vi "GET.vi"(6 "timeout (10000)":i32=10000, 7 "output file":path=path "", 8 "error in (no error)":errorcluster, 10 "url":string, 11 "HTTP Client Base in":refnum<class "HTTP Client Base.lvclass">) -> (0 "error out":errorcluster, 1 "body":string, 2 "headers":string, 3 "HTTP Client Base out":refnum<class "HTTP Client Base.lvclass">)   [LabVIEW 2021, in "HTTP Client Base.lvclass"]
uses:
  HTTP Client Base.lvclass
  HTTP Client Base.lvclass/HTTP Client Base.ctl
  <vilib>/httpClient/LabVIEWHTTPClient.lvlib
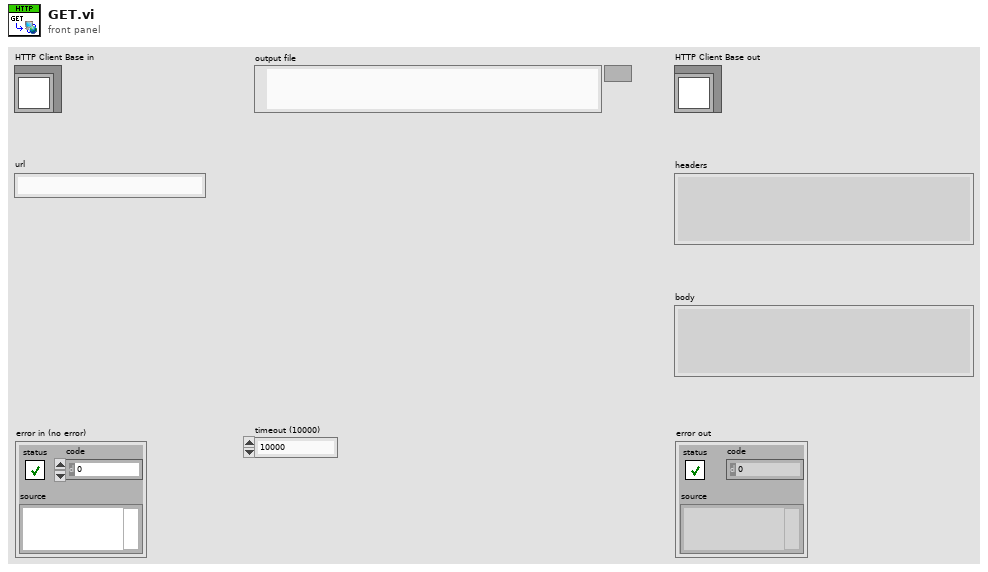
[diagram p1: front panel]
types:
  T1 = typedef "LabVIEWHTTPClient.lvlib/ClientHandle.ctl" = refnum<k1>
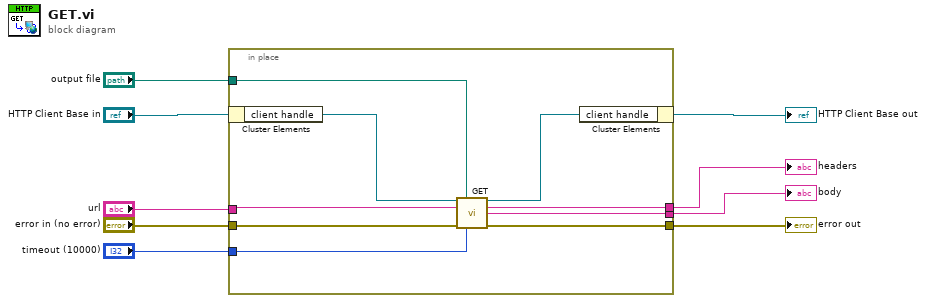
[diagram p0: block diagram]
diagram:
  n1 = in-place {
    in-place-border: [w12] -> w8
    in-place-border: "url" -> [w15]
    in-place-border: [w10] -> w1
    in-place-border: [w11] -> w2
    in-place-border: "error in (no error)" -> [w14]
    in-place-border: "output file" -> [w16]
    in-place-border: "timeout (10000)" -> [w13]
    n2 = in-place-cluster #1("HTTP Client Base in") -> ("client handle"=w18:T1)
    n3 = call <vilib>:"GET.vi"("client handle"=w18, "output file"=w16, "url"=w15, "error in (no error)"=w14, "timeout (10000)"=w13) -> ("client handle out"=w17:T1, "headers"=w11:string, "body"=w10:string, "error out"=w12:errorcluster)  [unwired: 7 in]
    n4 = in-place-cluster #1("client handle"=w17) -> (→"HTTP Client Base out":refnum<class "HTTP Client Base.lvclass">)
  }
  "error out" <- w8
  "headers" <- w2
  "body" <- w1
